vi "Control Panel.vi"(8 "error in (no error)":errorcluster, 11 "Level Meter.lvclass":refnum<class "Level Meter.lvclass">) -> (0 "error out":errorcluster, 3 "Magnet.lvclass out":refnum<class "Level Meter.lvclass">)   [LabVIEW 2009, in "Level Meter.lvclass"]
uses:
  Level Meter.lvclass
  Cryogen Levels.ctl
  Utility Classes/InstrPtr/InstrPtr.lvclass
  Global/Relative Sound Files.vi
  Level Meter.lvclass/Level Meter.ctl
  File IO/File IO.lvclass
panel:
  out "log update?":bool
  out "Alarm":bool
  out "*ilm200":T1
  in  "Display last":dbl[unit]=600.0
  out "TX graph":T2(graph)
  in  "Update interval":dbl[unit]=0.1
  in  "Internal UI Refresh":bool
  out "done?":bool
  out "Heliters":dbl caption="LHe Liters" format="%.3f"
  in  "Fast? He":bool
  in  "warningcontN":T3={"alarmliqN"=90.0, "warn?N"=FALSE, "lessthan?N"=FALSE}
  in  "warningcontHe":T4={"alarmliqHe"=85.0, "warn?He"=FALSE, "lessthan?He"=FALSE}
  out "Cryogen Levels":T5 min=-1.0 max=100.0 scale=0.0..100.0
  out "helium":T6 caption="Helium"
  out "nitrogen":cluster{"fillN?":bool, "lowN?":bool} caption="Nitrogen"
  out "shutdown":bool caption="Shut Down"
  out "active":bool
  out "working":bool caption="Working"
  out "ready?":bool
  in  "Refresh":bool
  in  "endprgm":bool
  # "Magnet Control Program"
  # "Helium"
  # "Cryogen Levels"
  # "Warning"
  # "Nitrogen"
  # "L"
  # "He Sample Rate"
  # "Slow"
  # "Fast"
  # "Off"
  # "On"
  # "Greater"
  # "Less"
  # "Off"
  # "On"
  # "Greater"
  # "Less"
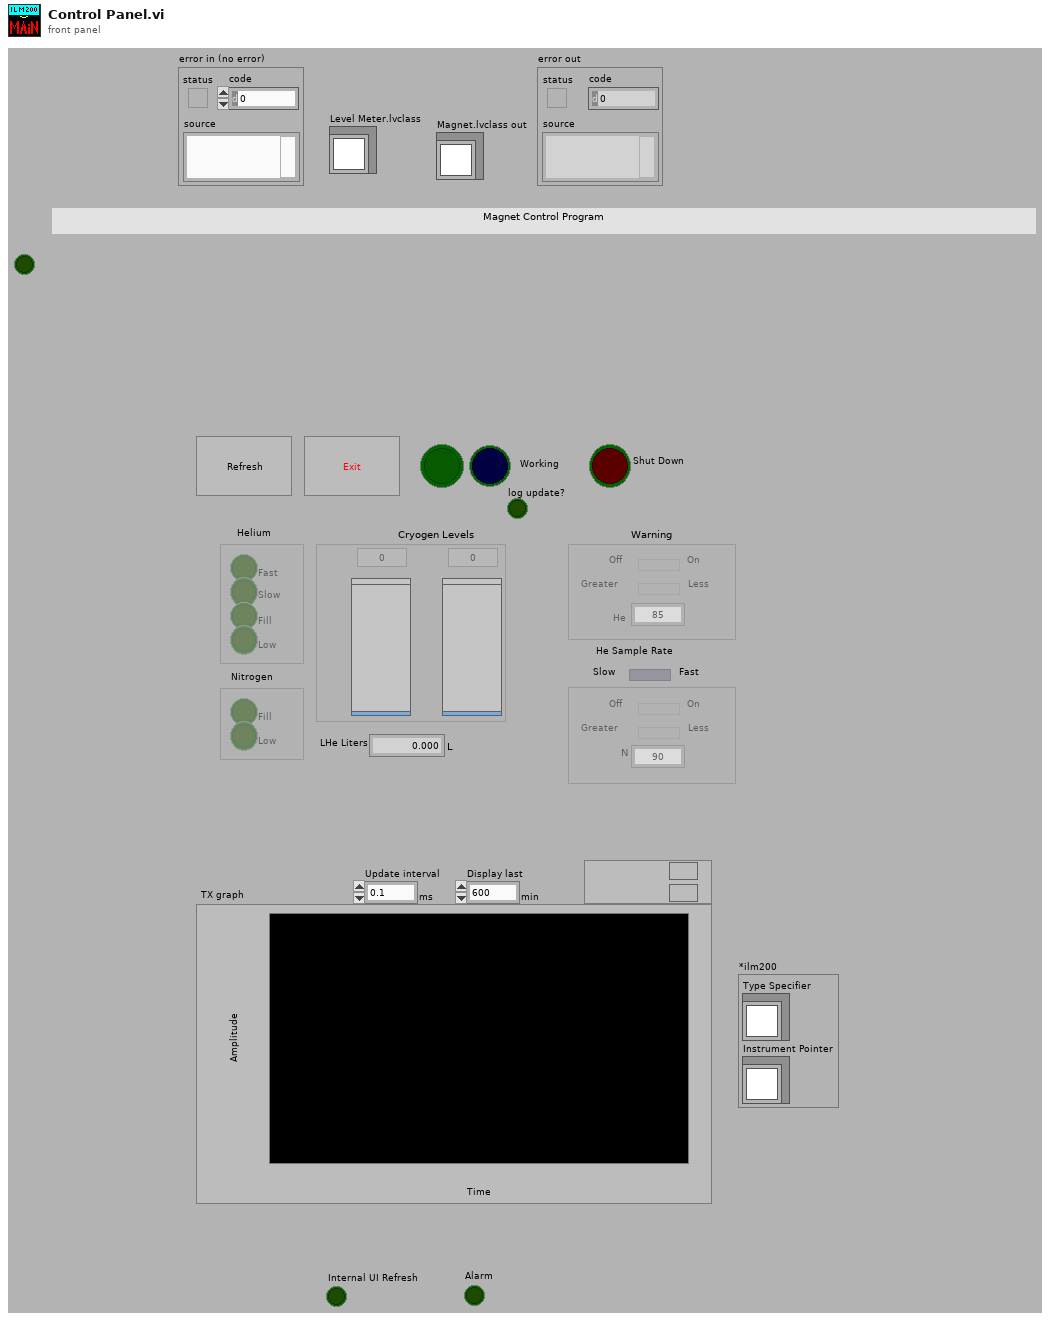
[diagram p1: front panel]
types:
  T1 = cluster{"Type Specifier":refnum<class "Level Meter.lvclass">, "Instrument Pointer":refnum<class "InstrPtr.lvclass">}
  T2 = cluster{"Data Points":cluster{"t":timestamp, "x":dbl}[]}[]
  T3 = cluster{"alarmliqN":dbl, "warn?N":bool, "lessthan?N":bool}
  T4 = cluster{"alarmliqHe":dbl, "warn?He":bool, "lessthan?He":bool}
  T5 = typedef "Level Meter.lvclass/Cryogen Levels.ctl" = dbl[]
  T6 = cluster{"fastHe?":bool, "slowHe?":bool, "fillHe?":bool, "lowHe?":bool}
  T7 = typedef "Readable.lvclass/TX Graph.ctl" = cluster{"Data Points":cluster{"t":timestamp, "x":dbl}[]}[]
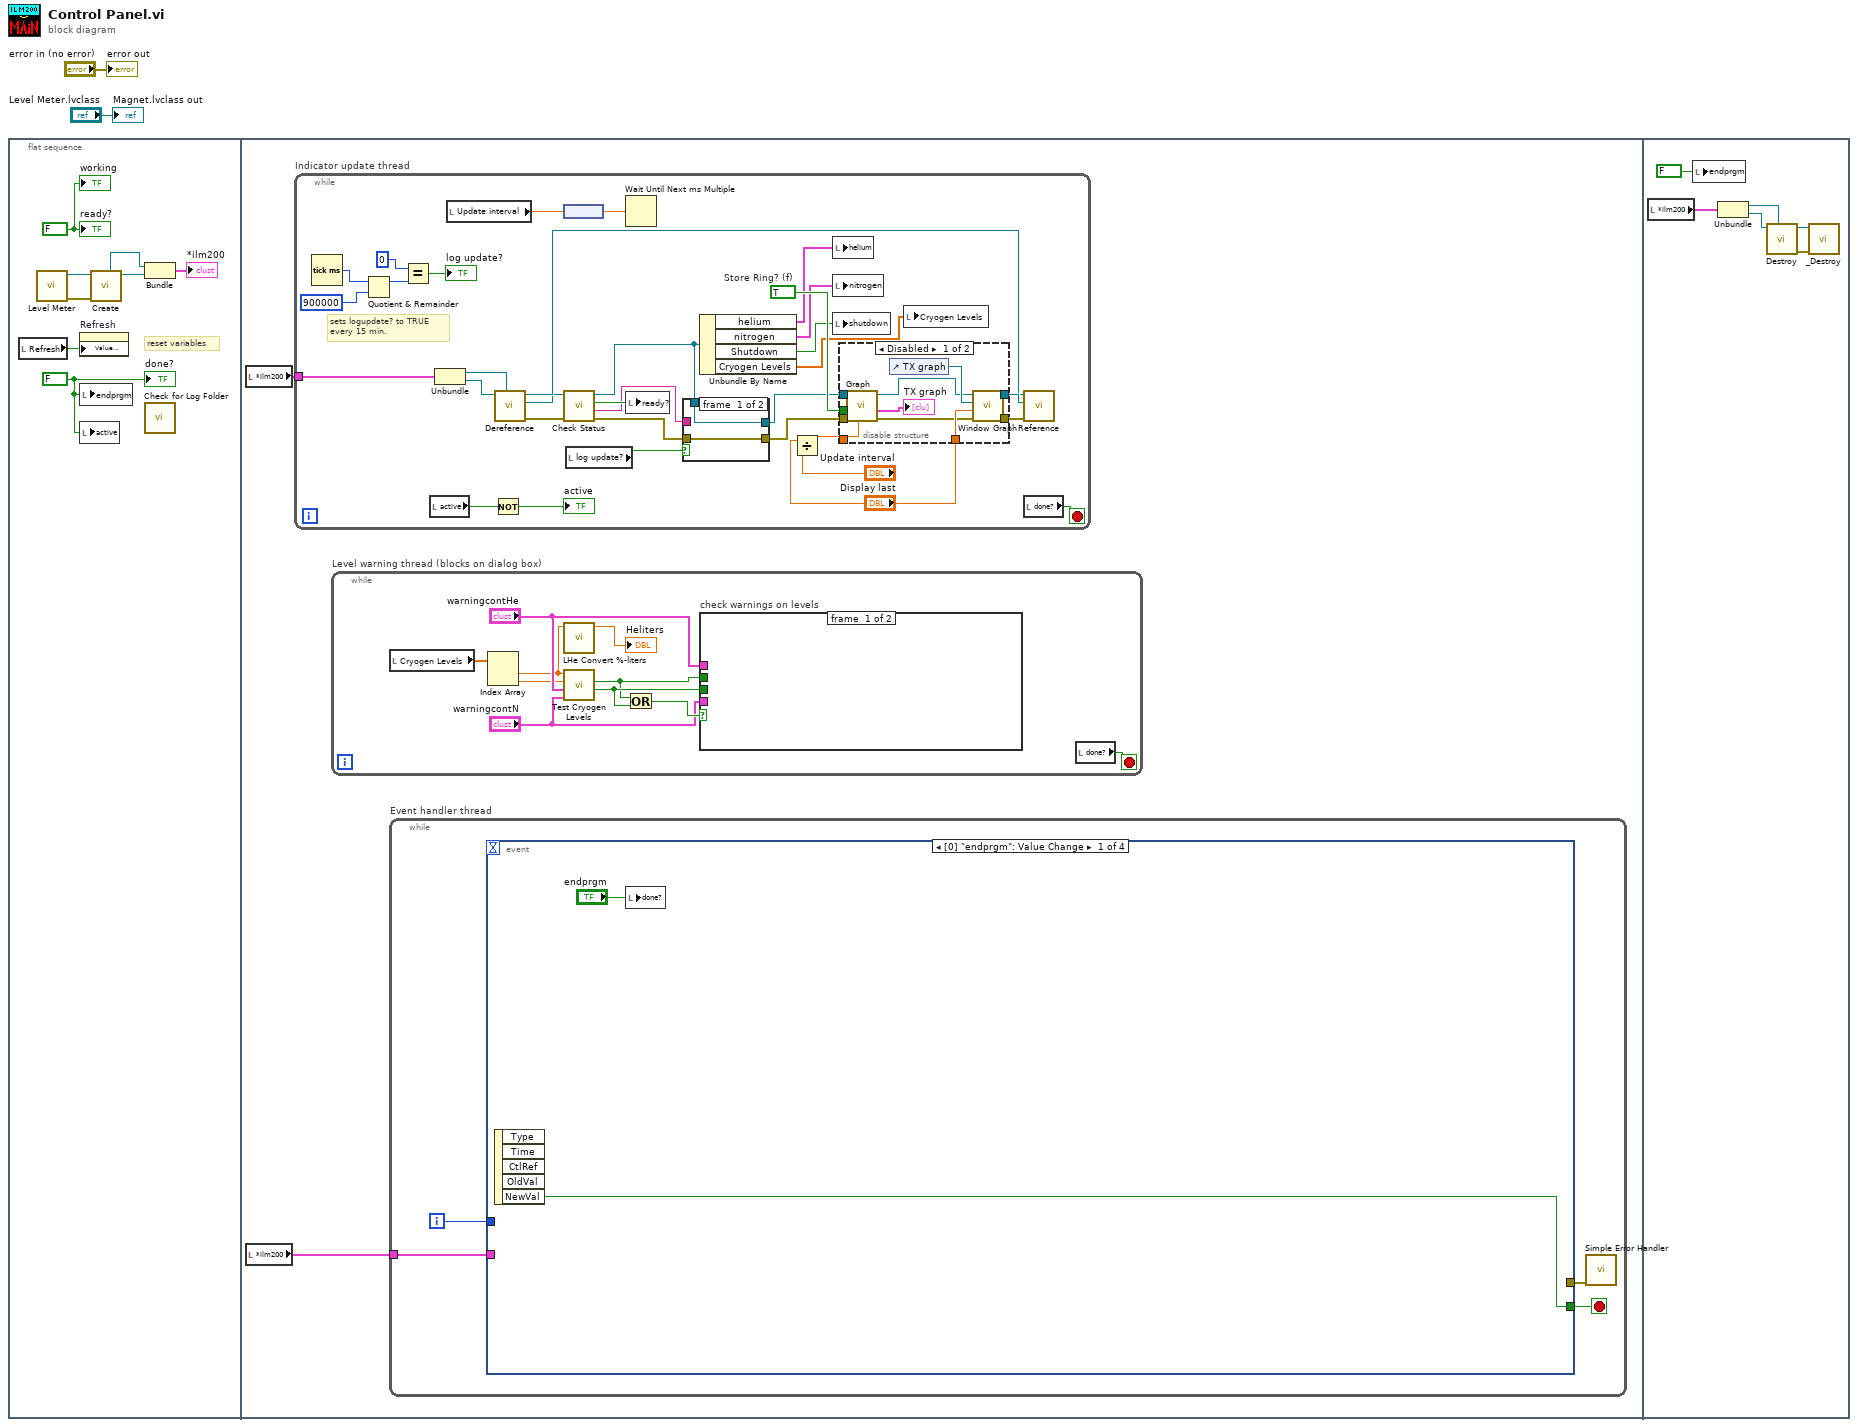
[diagram p0: block diagram]
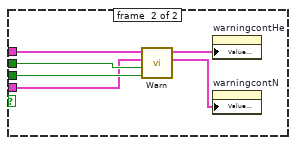
[diagram p2: hidden frame]
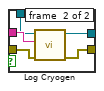
[diagram p3: hidden frame]
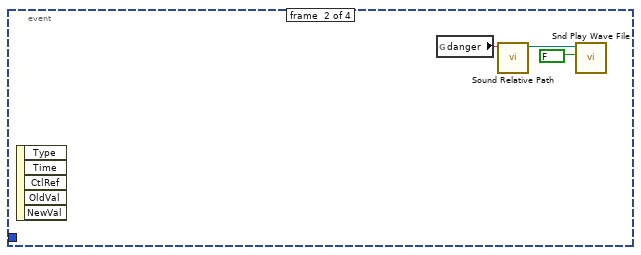
[diagram p5: hidden frame]
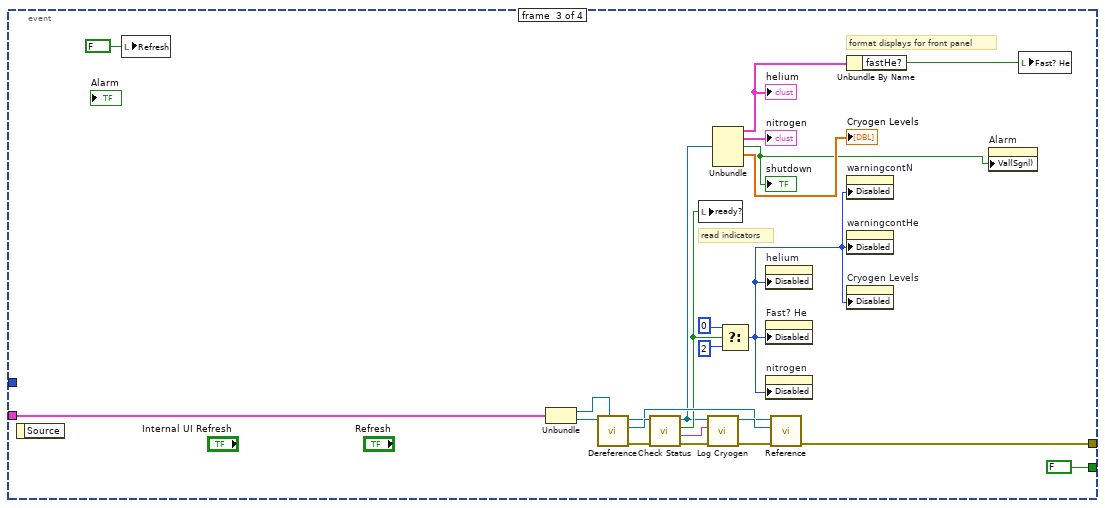
[diagram p6: hidden frame]
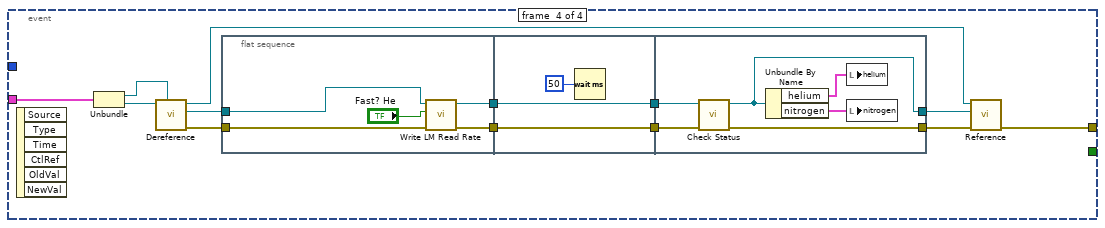
[diagram p7: hidden frame]
diagram:
  n1 = flat-sequence {
    frame #0 {
      w10 = FALSE
      w8 = FALSE
      # "reset variables"
      n2 = local read "Refresh"() -> (w9:bool)
      n3 = call "Level Meter.vi"() -> ("error out"=w6:errorcluster, "Level Meter out"=w7:refnum<class "Level Meter.lvclass">)  [unwired: 10 in]
      n4 = property on="Refresh" class="Bool (strict)"("Value (Signaling)"=w9) -> ()  [unwired: 2 in, 2 out]
      n5 = local write "endprgm"(w8) -> ()
      n6 = local write "active"(w8) -> ()
      n7 = call "Create.vi"("error in (no error)"=w6, "Instrument in"=w7) -> ("Instrument Pointer"=w5:refnum<class "InstrPtr.lvclass">, "Type Specifier"=w4:refnum<class "Level Meter.lvclass">)  [unwired: 7 in, 1 out]
      n8 = Bundle("Type Specifier"=w4, "Instrument Pointer"=w5) -> (→"*ilm200":T1)  [unwired: 1 in]
      n9 = call "Check for Log Folder.vi"() -> ()  [unwired: 1 out]
      "ready?" <- w10
      "working" <- w10
      "done?" <- w8
    }
    frame #1 {
      n10 = local read "*ilm200"() -> (w12:T1)
      n11 = local read "*ilm200"() -> (w11:T1)
      n12 = while "Indicator update thread" {
        tunnel: w12 -> [w51]
        stop <- w40 stop-if-true
        w61 = TRUE  # Store Ring? (f)
        # "sets logupdate? to TRUE\nevery 15 min."
        n13 = Tick Count (ms)() -> (millisecond timer value=w32:u32)
        n14 = Quotient & Remainder(x=w32, y=u32 900000) -> (x-y*floor(x/y)=w30:u32)  [unwired: 1 out]
        n15 = Equal?(x=0, y=w30) -> (x = y?=→"log update?":bool)
        n16 = local read "active"() -> (w54:bool)
        n17 = Unbundle(w51) -> ("Type Specifier"=w52:refnum<class "Level Meter.lvclass">, "Instrument Pointer"=w53:refnum<class "InstrPtr.lvclass">)
        n18 = local read "Update interval"() -> (w56:dbl[unit])
        n19 = Not(x=w54) -> (.not. x?=→"active":bool)
        n20 = call "Dereference.vi"("Type Specifier"=w52, "InstrPtr"=w53) -> ("error out"=w42:errorcluster, "Instrument out"=w43:refnum<class "Level Meter.lvclass">, "InstrPtr out"=w49:refnum<class "InstrPtr.lvclass">)  [unwired: 7 in]
        n21 = node(w56) -> (w60:dbl)
        n22 = call-dynamic "Check Status.vi"("error in (no error)"=w42, "Level Meter in"=w43) -> ("error out"=w39:errorcluster, "Status"=w38:string, "On?"=w41:bool, "Level Meter out"=w35:refnum<class "Level Meter.lvclass">)  [unwired: 6 in]
        n23 = local read "log update?"() -> (w36:bool)
        n24 = Wait Until Next ms Multiple(millisecond multiple=w60) -> ()  [unwired: 1 out]
        n25 = local write "ready?"(w41) -> ()
        n26 = case shown="True" w36 {
          tunnel: w39 -> [w62 w68]
          tunnel: [w62 w67] -> w34
          tunnel: w38 -> [_ w66]
          tunnel: w35 -> [w63 w65]
          tunnel: [w63 w64] -> w37
          frame #0 {
          }
          frame #1 {
            n27 = call-dynamic "Log Cryogen.vi"("error in (no error)"=w68, "Status string"=w66, "Level Meter in"=w65) -> ("error out"=w67:errorcluster, "Level Meter out"=w64:refnum<class "Level Meter.lvclass">)  [unwired: 7 in]
          }
        }
        n28 = Unbundle By Name(w35) -> ("helium"=w44:T6, "nitrogen"=w46:cluster{"fillN?":bool, "lowN?":bool}, "Shutdown"=w45:bool, "Cryogen Levels"=w47:T5)
        n29 = Divide(x="Display last", y="Update interval") -> (x/y=w58:dbl)
        n30 = local write "helium"(w44) -> ()
        n31 = local write "nitrogen"(w46) -> ()
        n32 = local write "shutdown"(w45) -> ()
        n33 = disable-structure shown="Disabled" {
          disable-tunnel: w61 -> [w79 _]
          disable-tunnel: w58 -> [w77 _]
          disable-tunnel: "Display last" -> [w76 _]
          disable-tunnel: w37 -> [w72 w81]
          disable-tunnel: w34 -> [w71 w80]
          disable-tunnel: [w70 w81] -> w50
          disable-tunnel: [w69 w80] -> w48
          frame #0 {
            n34 = call-dynamic "Graph.vi"("Ring size (points) (1024)"=w77, "error in (no error)"=w71, "Store Ring? (f)"=w79, "Readable in"=w72) -> ("error out"=w73:errorcluster, "Ring Buffers"=→"TX graph":T7, "Readable out"=w74:refnum<class "Level Meter.lvclass">)  [unwired: 3 in, 2 out]
            n35 = control-ref of="TX graph"() -> (w75:refnum<vi>)
            n36 = call-dynamic "Window Graph.vi"("error in (no error)"=w73, "Window"=w76, "Graph ref"=w75, "Readable in"=w74) -> ("error out"=w69:errorcluster, "Readable out"=w70:refnum<class "Level Meter.lvclass">)  [unwired: 6 in]
          }
          frame #1 {
          }
        }
        n37 = local write "Cryogen Levels"(w47) -> ()
        n38 = call "Reference.vi"("error in (no error)"=w48, "Instrument"=w50, "InstrPtr in"=w49) -> ()  [unwired: 8 in, 1 out]
        n39 = local read "done?"() -> (w40:bool)
      }
      n40 = while "Level warning thread (blocks on dialog box)" {
        stop <- w13 stop-if-true
        n41 = local read "Cryogen Levels"() -> (w14:T5)
        n42 = Index Array(array=w14) -> (element #1=w16:dbl, element #2=w15:dbl)  [unwired: 2 in]
        n43 = call "LHe Convert %-liters.vi"("%"=w16) -> ("Lout"=→"Heliters":dbl)  [unwired: 1 in, 9 out]
        n44 = call "Test Cryogen Levels.vi"("warningcontN"="warningcontN", "warningcontHe"="warningcontHe", "LNlevel"=w15, "LHelevel"=w16) -> ("warnN"=w21:bool, "warnHe"=w20:bool)  [unwired: 1 in, 5 out]
        n45 = Or(x=w20, y=w21) -> (x .or. y?=w19:bool)
        n46 = case "check warnings on levels" shown="True" w19 {
          tunnel: w20 -> [_ w28]
          tunnel: w21 -> [_ w27]
          tunnel: "warningcontHe" -> [_ w26]
          tunnel: "warningcontN" -> [_ w25]
          frame #0 {
          }
          frame #1 {
            n47 = call "Warn.vi"("NwarnIN"=w27, "HwarnIN"=w28, "warncontN"=w25, "warncontHe"=w26) -> ("warnNOUT"=w24:T3, "warnHeOUT"=w23:T4)  [unwired: 1 in, 5 out]
            n48 = property on="warningcontHe" class="Clust (strict)"("Value (Signaling)"=w23) -> ()  [unwired: 2 in, 2 out]
            n49 = property on="warningcontN" class="Cluster (strict)"("Value (Signaling)"=w24) -> ()  [unwired: 2 in, 2 out]
          }
        }
        n50 = local read "done?"() -> (w13:bool)
      }
      n51 = while "Event handler thread" {
        tunnel: w11 -> [w83]
        i -> [w84]
        stop <- w85 stop-if-true
        n52 = event shown="[0] \"endprgm\": Value Change" {
          selector: _ -> [_ _ _ _]
          dyn-events: _ -> [_ _ _ _]
          timeout: _ -> [_ _ _ _]
          tunnel: [w87 _ FALSE _] -> w85
          tunnel: w84 -> [_ _ _ _]
          tunnel: w83 -> [_ _ w109 w124]
          tunnel: [_ _ w104 w114] -> w82
          event #0 {
            n53 = event-data() -> ("NewVal"=w87:bool)  [unwired: 5 out]
            n54 = local write "done?"("endprgm") -> ()
          }
          event #1 {
            n55 = event-data() -> ()  [unwired: 6 out]
            n56 = global read "Relative Sound Files.vi" "danger"() -> (w89:string)
            n57 = call "Sound Relative Path.vi"("Sound"=w89) -> ("Relative Path"=w88:path)  [unwired: 10 in]
            n58 = call <vilib>:"Snd Play Wave File.vi"("wait until finish (T)"=FALSE, "wave file path"=w88) -> ()  [unwired: 1 in, 9 out]
          }
          event #2 {
            # "format displays for front panel"
            # "read indicators"
            n59 = event-data() -> ()  [unwired: 2 out]
            n60 = local write "Refresh"(FALSE) -> ()
            n61 = Unbundle(w109) -> ("Type Specifier"=w111:refnum<class "Level Meter.lvclass">, "Instrument Pointer"=w110:refnum<class "InstrPtr.lvclass">)
            n62 = call "Dereference.vi"("Type Specifier"=w111, "InstrPtr"=w110) -> ("error out"=w103:errorcluster, "Instrument out"=w108:refnum<class "Level Meter.lvclass">, "InstrPtr out"=w106:refnum<class "InstrPtr.lvclass">)  [unwired: 7 in]
            n63 = call-dynamic "Check Status.vi"("error in (no error)"=w103, "Level Meter in"=w108) -> ("error out"=w93:errorcluster, "Status"=w92:string, "On?"=w99:bool, "Level Meter out"=w94:refnum<class "Level Meter.lvclass">)  [unwired: 6 in]
            n64 = local write "ready?"(w99) -> ()
            n65 = call-dynamic "Log Cryogen.vi"("error in (no error)"=w93, "Status string"=w92, "Level Meter in"=w94) -> ("error out"=w105:errorcluster, "Level Meter out"=w107:refnum<class "Level Meter.lvclass">)  [unwired: 7 in]
            n66 = Unbundle(w94) -> (w96:T6, →"nitrogen":cluster{"fillN?":bool, "lowN?":bool}, w91:bool, →"Cryogen Levels":T5)  [unwired: 1 out]
            "helium" <- w96
            "shutdown" <- w91
            n67 = Select(t=0, s=w99, f=2) -> (s? t:f=w100:i32)
            n68 = property on="helium" class="Cluster (strict)"("Disabled"=w100) -> ()  [unwired: 2 in, 2 out]
            n69 = property on="Fast? He" class="Boolean (strict)"("Disabled"=w100) -> ()  [unwired: 2 in, 2 out]
            n70 = property on="nitrogen" class="Cluster (strict)"("Disabled"=w100) -> ()  [unwired: 2 in, 2 out]
            n71 = call "Reference.vi"("error in (no error)"=w105, "Instrument"=w107, "InstrPtr in"=w106) -> ("error out"=w104:errorcluster)  [unwired: 8 in]
            n72 = Unbundle By Name(w96) -> ("fastHe?"=w95:bool)
            n73 = property on="warningcontN" class="Cluster (strict)"("Disabled"=w100) -> ()  [unwired: 2 in, 2 out]
            n74 = property on="warningcontHe" class="Clust (strict)"("Disabled"=w100) -> ()  [unwired: 2 in, 2 out]
            n75 = property on="Cryogen Levels" class="Arr (strict)"("Disabled"=w100) -> ()  [unwired: 2 in, 2 out]
            n76 = property on="Alarm" class="Bool (strict)"("Val(Sgnl)"=w91) -> ()  [unwired: 2 in, 2 out]
            n77 = local write "Fast? He"(w95) -> ()
          }
          event #3 {
            n78 = event-data() -> ()  [unwired: 7 out]
            n79 = Unbundle(w124) -> ("Type Specifier"=w126:refnum<class "Level Meter.lvclass">, "Instrument Pointer"=w125:refnum<class "InstrPtr.lvclass">)
            n80 = call "Dereference.vi"("Type Specifier"=w126, "InstrPtr"=w125) -> ("error out"=w118:errorcluster, "Instrument out"=w119:refnum<class "Level Meter.lvclass">, "InstrPtr out"=w123:refnum<class "InstrPtr.lvclass">)  [unwired: 7 in]
            n81 = flat-sequence {
              tunnel: [w130] -> w121
              tunnel: w119 -> [w129]
              tunnel: w118 -> [w128]
              tunnel: [w127] -> w116
              tunnel: w121 -> [w133]
              tunnel: [w133] -> w120
              tunnel: [w132] -> w117
              tunnel: w116 -> [w132]
              tunnel: [w138] -> w122
              tunnel: w120 -> [w137]
              tunnel: w117 -> [w136]
              tunnel: [w135] -> w115
              frame #0 {
                n82 = call-dynamic "Write LM Read Rate.vi"("error in (no error)"=w128, "Fast?"="Fast? He", "Level Meter in"=w129) -> ("error out"=w127:errorcluster, "Level Meter out"=w130:refnum<class "Level Meter.lvclass">)  [unwired: 7 in]
              }
              frame #1 {
                n83 = Wait (ms)(milliseconds to wait=50) -> ()  [unwired: 1 out]
              }
              frame #2 {
                n84 = call-dynamic "Check Status.vi"("error in (no error)"=w136, "Level Meter in"=w137) -> ("error out"=w135:errorcluster, "Level Meter out"=w138:refnum<class "Level Meter.lvclass">)  [unwired: 6 in, 2 out]
                n85 = Unbundle By Name(w138) -> ("helium"=w140:T6, "nitrogen"=w139:cluster{"fillN?":bool, "lowN?":bool})
                n86 = local write "helium"(w140) -> ()
                n87 = local write "nitrogen"(w139) -> ()
              }
            }
            n88 = call "Reference.vi"("error in (no error)"=w115, "Instrument"=w122, "InstrPtr in"=w123) -> ("error out"=w114:errorcluster)  [unwired: 8 in]
          }
        }
        n89 = call <vilib>:"Simple Error Handler.vi"("error in (no error)"=w82) -> ()  [unwired: 4 in, 5 out]
      }
    }
    frame #2 {
      n90 = local read "*ilm200"() -> (w143:T1)
      n91 = local write "endprgm"(FALSE) -> ()
      n92 = Unbundle(w143) -> ("Type Specifier"=w142:refnum<class "Level Meter.lvclass">, "Instrument Pointer"=w141:refnum<class "InstrPtr.lvclass">)
      n93 = call "Destroy.vi"("Type Specifier"=w142, "InstrPtr in"=w141) -> ("error out"=w145:errorcluster, "final Instrument"=w144:refnum<class "Level Meter.lvclass">)  [unwired: 8 in]
      n94 = call-dynamic "_Destroy.vi"("error in (no error)"=w145, "Instrument in"=w144) -> ()  [unwired: 9 in, 1 out]
    }
  }
  "Magnet.lvclass out" <- "Level Meter.lvclass"
  "error out" <- "error in (no error)"
